vi "Display_drawScene.vi"(8 "error in":errorcluster, 11 "DisplayData":T1) -> (0 "error out":errorcluster, 3 "DisplayData 2":T1)   [LabVIEW 2017]
uses:
  Display_data.ctl
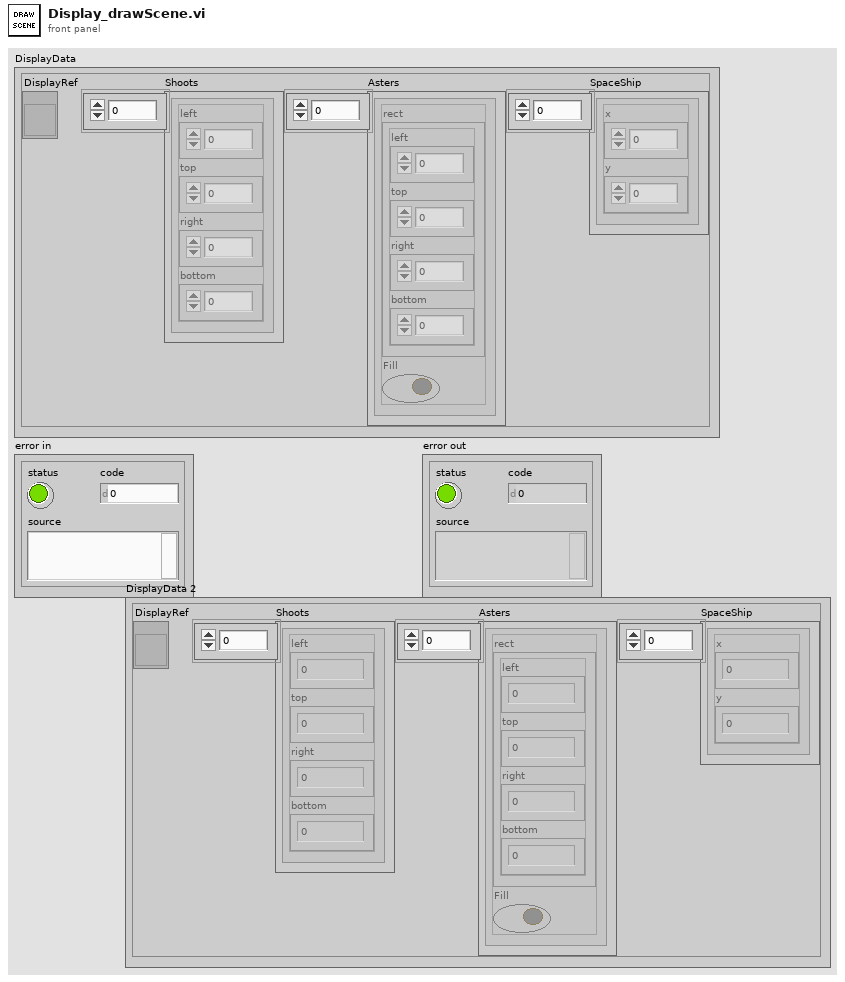
[diagram p1: front panel]
types:
  T1 = typedef "Display_data.ctl" = cluster{"DisplayRef":refnum<vi>, "Shoots":cluster{"left":i16, "top":i16, "right":i16, "bottom":i16}[], "Asters":cluster{"rect":cluster{"left":i16, "top":i16, "right":i16, "bottom":i16}, "Fill":bool}[], "SpaceShip":cluster{"x":i16, "y":i16}[]}
  T2 = cluster{"rect":cluster{"left":i16, "top":i16, "right":i16, "bottom":i16}, "Fill":bool}[]
  T3 = cluster{"left":i16, "top":i16, "right":i16, "bottom":i16}
  T4 = cluster{"left":i16, "top":i16, "right":i16, "bottom":i16}[]
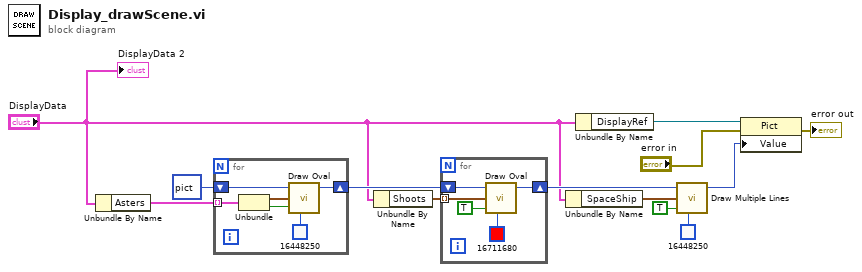
[diagram p0: block diagram]
diagram:
  n1 = Unbundle By Name("DisplayData") -> ("Asters"=w13:T2)
  n2 = for {
    tunnel: w13 -> [w16] mode=indexing
    shift-right: [w14] -> w11
    shift-left: picture data[5B] ("picture") -> [w15]
    n3 = Unbundle(w16) -> ("rect"=w17:T3, "Fill"=w18:bool)
    n4 = call <vilib>:"Draw Oval.vi"("picture"=w15, "rect"=w17, "fill?(F)"=w18, "color(black)"=u32 16448250) -> ("new picture"=w14:picture)  [unwired: 5 in]
  }
  n5 = Unbundle By Name("DisplayData") -> ("Shoots"=w10:T4)
  n6 = for {
    shift-right: [w21] -> w7
    shift-left: w11 -> [w22]
    tunnel: w10 -> [w20] mode=indexing
    n7 = call <vilib>:"Draw Oval.vi"("picture"=w22, "rect"=w20, "fill?(F)"=TRUE, "color(black)"=u32 16711680) -> ("new picture"=w21:picture)  [unwired: 5 in]
  }
  n8 = Unbundle By Name("DisplayData") -> ("SpaceShip"=w6:cluster{"x":i16, "y":i16}[])
  n9 = Unbundle By Name("DisplayData") -> ("DisplayRef"=w4:refnum<vi>)
  n10 = call <vilib>:"Draw Multiple Lines.vi"("picture"=w7, "line endpoints"=w6, "fill?(F)"=TRUE, "color(black)"=u32 16448250) -> ("new picture"=w3:picture)  [unwired: 5 in]
  n11 = property class="Pict"(reference=w4, error in="error in", "Value"=w3) -> (error out=→"error out":errorcluster)  [unwired: 1 out]
  "DisplayData 2" <- "DisplayData"
